vi "TrueOrFalse.vi"(8 "error out":errorcluster, 11 "布尔":bool) -> (0 "error out 2":errorcluster caption="error out")   [LabVIEW 2014]
uses:
  <vilib>/addons/database/Connection.llb/DB Tools Open Connec (String).vi
  <vilib>/addons/database/Connection.llb/Conn Execute.vi
  <vilib>/addons/database/Recordset.llb/Rec Destroy - Connection.vi
  <vilib>/addons/database/NI_Database_API.lvlib
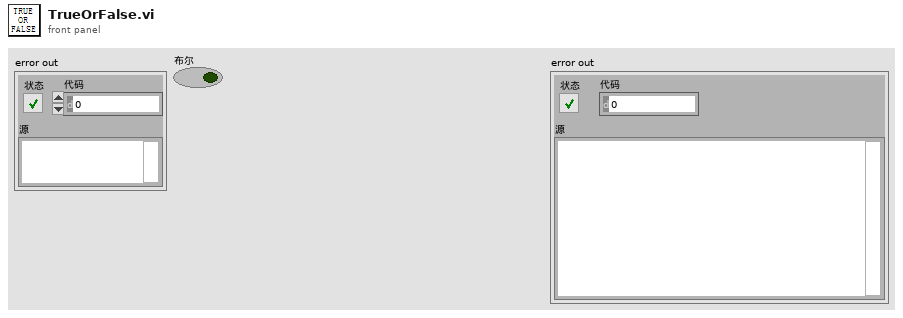
[diagram p1: front panel]
types:
  T1 = typedef "NI_Database_API.lvlib/Conn ObjectReference.ctl" = refnum<k1>
  T2 = typedef "NI_Database_API.lvlib/Rec ObjectReference.ctl" = refnum<k1>
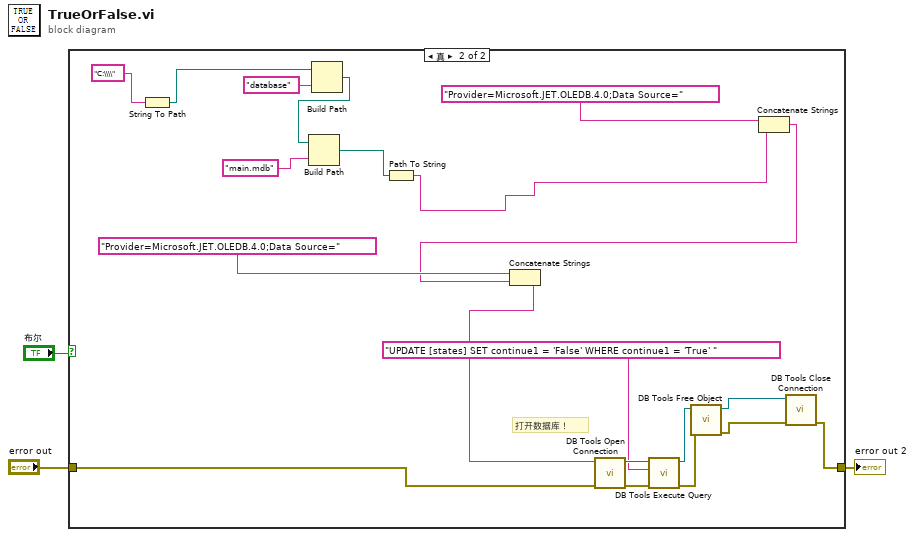
[diagram p0: block diagram]
diagram:
  n1 = case shown="真" "布尔" {
    tunnel: "error out" -> [w4 w7]
    tunnel: [w4 w15] -> w1
    frame False {
    }
    frame True {
      # "打开数据库！"
      n2 = String To Path(string="C:\\\\") -> (path=w5:path)
      n3 = Build Path(base path=w5, name or relative path="database" ("名称或相对路径")) -> (appended path=w13:path)
      n4 = Build Path(base path=w13, name or relative path="main.mdb" ("名称或相对路径")) -> (appended path=w14:path)
      n5 = Path To String(path=w14) -> (string=w9:string)
      n6 = Concatenate Strings("Provider=Microsoft.JET.OLEDB.4.0;Data Source=", w9) -> (w8:string)
      n7 = Concatenate Strings("Provider=Microsoft.JET.OLEDB.4.0;Data Source=", w8) -> (w23:string)
      n8 = call-poly <vilib>:"DB Tools Open Connection.vi"("error in (no error)"=w7, "connection information"=w23) -> ("error out"=w21:errorcluster, "connection reference"=w22:T1)  [unwired: 6 in]
      n9 = call-poly <vilib>:"DB Tools Execute Query.vi"("error in (no error)"=w21, "SQL query"="UPDATE [states] SET continue1 = 'False' WHERE continue1 = 'True' ", "connection reference"=w22) -> ("error out"=w16:errorcluster, "recordset reference"=w17:T2)  [unwired: 5 in]
      n10 = call-poly <vilib>:"DB Tools Free Object.vi"("error in (no error)"=w16, "recordset reference"=w17) -> ("error out"=w19:errorcluster, "connection reference"=w18:T1)  [unwired: 8 in]
      n11 = call <vilib>:"DB Tools Close Connection.vi"("error in (no error)"=w19, "connection reference"=w18) -> ("error out"=w15:errorcluster)  [unwired: 5 in]
    }
  }
  "error out 2" <- w1
